vi "HEAD.vi"(6 "timeout":i32=10000, 8 "error in":errorcluster, 10 "url":string, 11 "http-client in":refnum<class "basic-http-client.lvclass">) -> (0 "error out":errorcluster, 2 "response":refnum<class "response.lvclass">, 3 "http-client out":refnum<class "basic-http-client.lvclass">)   [LabVIEW 2020, in "http.lvlib" / "basic-http-client.lvclass"]
uses:
  basic-http-client.lvclass
  response/response.lvclass
  basic-http-client.lvclass/basic-http-client.ctl
  <vilib>/httpClient/LabVIEWHTTPClient.lvlib
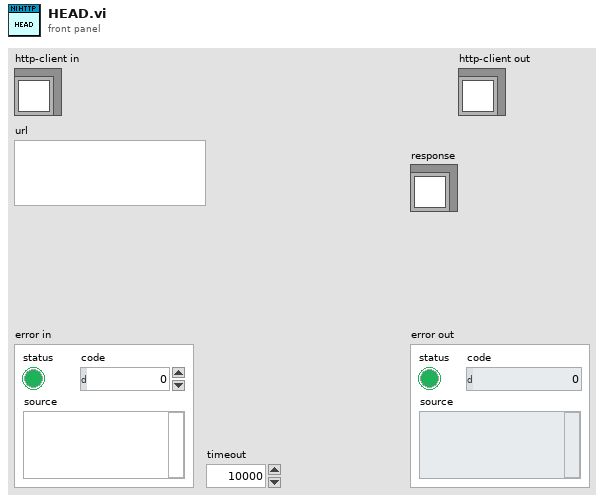
[diagram p1: front panel]
types:
  T1 = typedef "LabVIEWHTTPClient.lvlib/ClientHandle.ctl" = refnum<k1>
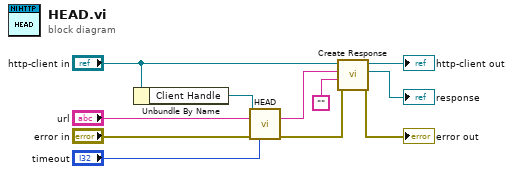
[diagram p0: block diagram]
diagram:
  n1 = Unbundle By Name("http-client in") -> ("Client Handle"=w7:T1)
  n2 = call <vilib>:"HEAD.vi"("client handle"=w7, "url"="url", "error in (no error)"="error in", "timeout (10000)"="timeout") -> ("headers"=w5:string, "error out"=w2:errorcluster)  [unwired: 9 in, 1 out]
  n3 = call-dynamic "Create Response.vi"("error in (no error)"=w2, "body"="", "headers"=w5, "http-client"="http-client in") -> ("error out"=→"error out":errorcluster, "response"=→"response":refnum<class "response.lvclass">, "http-client out"=→"http-client out":refnum<class "basic-http-client.lvclass">)  [unwired: 5 in]
